vi "Actor Core.vi"(8 "error in":errorcluster, 11 "Nested in":refnum<class "Contador.lvclass">) -> (0 "error out":errorcluster, 3 "Actor out":refnum<class "Actor.lvclass">)   [LabVIEW 2020, in "Contador.lvlib" / "Contador.lvclass"]
doc: "(<B>Filename</B>: Actor Framework.lvlib:Actor.lvclass:Actor Core.vi)\n\nReceives messages to the actor, reacts to them, and initiates any error handling that may shut the actor down.\n\nDescendant classes may override this VI to append parallel tasks for the actor to complete while it handles messages. Overrides use the Call Parent Method node."
uses:
  Contador.lvclass
  C:/Program Files (x86)/National Instruments/LabVIEW 2020/vi.lib/ActorFramework/Actor/Actor.lvclass
  <vilib>/ActorFramework/Actor/Actor.lvclass
  ACQ Contador/ACQ Contador/ACQ Contador.lvclass
  Contador.lvclass/Contador.ctl
  <vilib>/ActorFramework/Actor/Actor.lvclass/Actor.ctl
  <vilib>/ActorFramework/Message Enqueuer/Message Enqueuer.lvclass/Message Enqueuer.ctl
  Contador Messages/Start Stop Msg/Start Stop Msg.lvclass/Start Stop Msg.ctl
  Contador Messages/Lim Superior Msg/Lim Superior Msg.lvclass/Lim Superior Msg.ctl
  Contador Messages/Lim Inferior Msg/Lim Inferior Msg.lvclass/Lim Inferior Msg.ctl
  Contador Messages/Save Enable Msg/Save Enable Msg.lvclass/Save Enable Msg.ctl
  Contador Messages/Path Msg/Path Msg.lvclass/Path Msg.ctl
  Contador Messages/File Type Msg/File Type Msg.lvclass/File Type Msg.ctl
  <vilib>/ActorFramework/Message Enqueuer/Init from Existing Queue.vi
  <vilib>/ActorFramework/Message Enqueuer/Enqueue.vi
  <vilib>/ActorFramework/Stop Msg/Stop Msg.lvclass
  C:/Program Files (x86)/National Instruments/LabVIEW 2020/vi.lib/ActorFramework/Message/Message.lvclass
  Contador Messages/Start Stop Msg/Start Stop Msg.lvclass
  Contador Messages/Lim Superior Msg/Lim Superior Msg.lvclass
  Contador Messages/Lim Inferior Msg/Lim Inferior Msg.lvclass
  Contador Messages/Save Enable Msg/Save Enable Msg.lvclass
  Contador Messages/Path Msg/Path Msg.lvclass
  Contador Messages/File Type Msg/File Type Msg.lvclass
  <vilib>/ActorFramework/Message Priority Queue/Priority Enqueue.vi
  <vilib>/ActorFramework/Message Enqueuer/Message Enqueuer.lvclass
panel:
  in  "File Type":u16(ring) items=["Text", "CSV"]
  in  "File Path":path
  in  "Save Button":bool
  in  "Stop":bool
  in  "Start":bool
  in  "Límite inferior":dbl
  in  "Límite superior":dbl
  out "Cuenta":bool[](array[boolean])
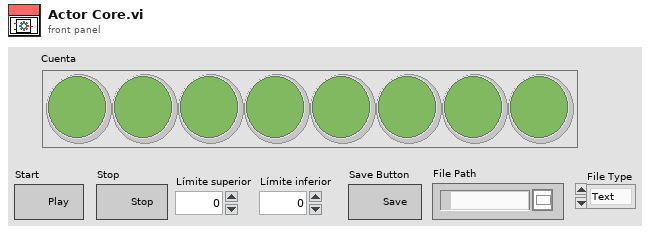
[diagram p1: front panel]
types:
  T1 = cluster{"Stop":refnum<user-event>, "Cuenta":refnum<user-event>}
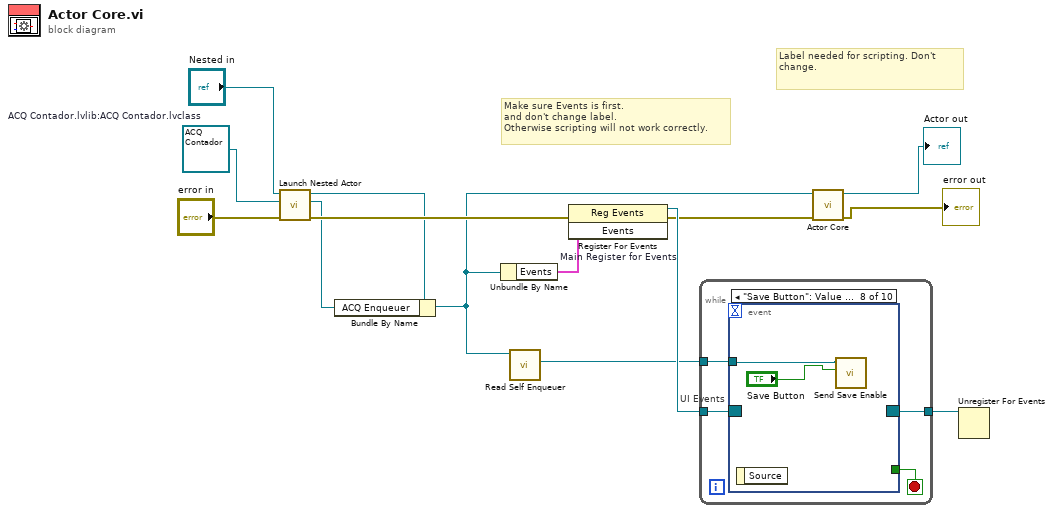
[diagram p0: block diagram]
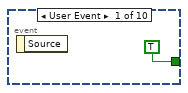
[diagram p2: hidden frame]
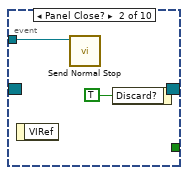
[diagram p3: hidden frame]
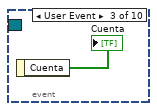
[diagram p4: hidden frame]
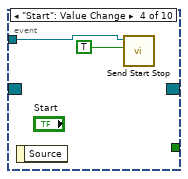
[diagram p5: hidden frame]
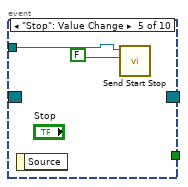
[diagram p6: hidden frame]
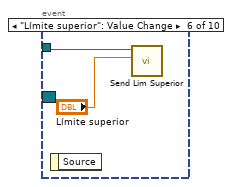
[diagram p7: hidden frame]
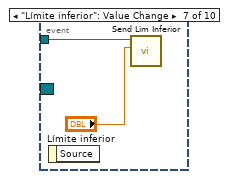
[diagram p8: hidden frame]
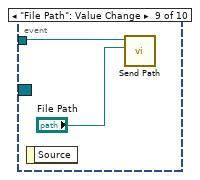
[diagram p9: hidden frame]
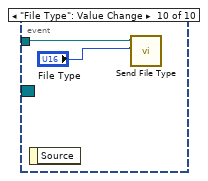
[diagram p10: hidden frame]
diagram:
  w3 = refnum<class "ACQ Contador.lvclass"> refnum  # ACQ Contador.lvlib:ACQ Contador.lvclass
  # "Label needed for scripting. Don't change."
  # "Make sure Events is first.\nand don't change label.\nOtherwise scripting will not work correctly."
  n1 = call <vilib>:"Launch Nested Actor.vi"("error in (no error)"="error in", "Nested Actor"=w3, "Caller Actor in"="Nested in") -> ("error out"=w9:errorcluster, "Nested Actor's Enqueuer"=w4:refnum<class "Message Enqueuer.lvclass">, "Caller Actor out"=w6:refnum<class "Contador.lvclass">)  [unwired: 6 in]
  n2 = Bundle By Name(cluster=w6, "ACQ Enqueuer"=w4) -> (w5:refnum<class "Contador.lvclass">)
  n3 = Unbundle By Name(w5) -> ("Events"=w12:T1)
  n4 = call <vilib>:"Read Self Enqueuer.vi"("Actor"=w5) -> ("Self Enqueuer"=w11:refnum<class "Message Enqueuer.lvclass">)  [unwired: 10 in]
  n5 = register-events "Main Register for Events"(error in=w9, w12) -> (reference out=w13:refnum<event-registration>, error out=w10:errorcluster)  [unwired: 1 in]
  n6 = while {
    tunnel: w13 -> [w18]
    tunnel: [w16] -> w1
    tunnel: w11 -> [w15]
    stop <- w17 stop-if-true
    n7 = event "UI Events" shown="[7] \"Save Button\": Value Change" {
      selector: w18 -> [_ _ _ _ _ _ _ _ _ _]
      dyn-events: [_ _ _ _ _ _ _ _ _ _] -> w16
      timeout: _ -> [_ _ _ _ _ _ _ _ _ _]
      tunnel: [TRUE _ _ _ _ _ _ _ _ _] -> w17
      tunnel: w15 -> [_ w20 _ w24 w26 w28 w30 w32 w34 w36]
      event User Event {
        n8 = event-data() -> ()  [unwired: 1 in, 1 out]
      }
      event Panel Close? {
        n9 = event-data() -> ()  [unwired: 1 in, 1 out]
        n10 = call <vilib>:"Send Normal Stop.vi"("Message Enqueuer"=w20) -> ()  [unwired: 10 in, 1 out]
        n11 = event-data("Discard?"=TRUE) -> ()  [unwired: 1 in, 1 out]
      }
      event User Event {
        n12 = event-data() -> ("Cuenta"=→"Cuenta":bool[])  [unwired: 1 in]
      }
      event "Start": Value Change {
        n13 = event-data() -> ()  [unwired: 1 in, 1 out]
        n14 = call "Send Start Stop.vi"("Start/Stop"=TRUE, "Message Enqueuer"=w24) -> ()  [unwired: 8 in, 2 out]
      }
      event "Stop": Value Change {
        n15 = event-data() -> ()  [unwired: 1 in, 1 out]
        n16 = call "Send Start Stop.vi"("Start/Stop"=FALSE, "Message Enqueuer"=w26) -> ()  [unwired: 8 in, 2 out]
      }
      event "Límite superior": Value Change {
        n17 = event-data() -> ()  [unwired: 1 in, 1 out]
        n18 = call "Send Lim Superior.vi"("MAX"="Límite superior", "Message Enqueuer"=w28) -> ()  [unwired: 8 in, 2 out]
      }
      event "Límite inferior": Value Change {
        n19 = event-data() -> ()  [unwired: 1 in, 1 out]
        n20 = call "Send Lim Inferior.vi"("MIN"="Límite inferior", "Message Enqueuer"=w30) -> ()  [unwired: 8 in, 2 out]
      }
      event "Save Button": Value Change {
        n21 = event-data() -> ()  [unwired: 1 in, 1 out]
        n22 = call "Send Save Enable.vi"("Save Enable"="Save Button", "Message Enqueuer"=w32) -> ()  [unwired: 8 in, 2 out]
      }
      event "File Path": Value Change {
        n23 = event-data() -> ()  [unwired: 1 in, 1 out]
        n24 = call "Send Path.vi"("Path"="File Path", "Message Enqueuer"=w34) -> ()  [unwired: 8 in, 2 out]
      }
      event "File Type": Value Change {
        n25 = event-data() -> ()  [unwired: 1 in, 1 out]
        n26 = call "Send File Type.vi"("File Type"="File Type", "Message Enqueuer"=w36) -> ()  [unwired: 8 in, 2 out]
      }
    }
  }
  n27 = call-parent "Actor Core.vi"("error in"=w10, "Actor in"=w5) -> ("error out"=→"error out":errorcluster, "Actor out"=→"Actor out":refnum<class "Actor.lvclass">)  [unwired: 8 in]
  n28 = Unregister For Events(event registration refnum=w1) -> ()  [unwired: 1 in, 1 out]
